vi "CloseConnection.vi"(8 "error in (no error)":errorcluster, 10 "timeout [ms]":i32=5000, 11 "Communicator in":refnum<class "Communicator.lvclass">) -> (0 "error out":errorcluster, 3 "Communicator out":refnum<class "Communicator.lvclass">)   [LabVIEW 2023, in "Communicator.lvclass"]
uses:
  Communicator.lvclass
  Communicator.lvclass/Communicator.ctl
  <vilib>/MediaMongrels Ltd/WebSockets/WebSockets/WebSocket Client/WebSocket Client.lvclass
panel:
  # "Connector Pane"
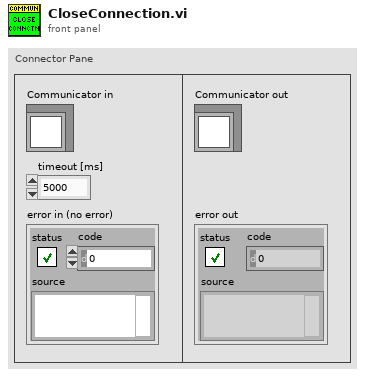
[diagram p1: front panel]
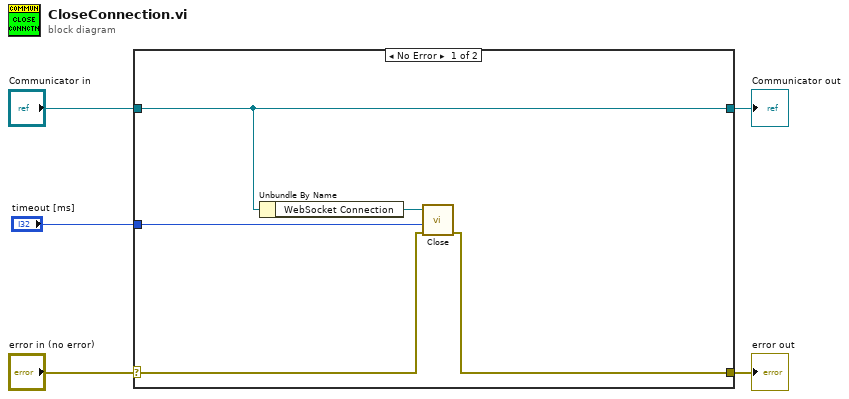
[diagram p0: block diagram]
diagram:
  n1 = case shown="No Error" "error in (no error)" {
    selector: "error in (no error)" -> [w10 w12]
    tunnel: [w9 w12] -> w4
    tunnel: [w8 w11] -> w2
    tunnel: "Communicator in" -> [w8 w11]
    tunnel: "timeout [ms]" -> [w6 _]
    frame No Error {
      n2 = Unbundle By Name(w8) -> ("WebSocket Connection"=w7:refnum<class "WebSocket Client.lvclass">)
      n3 = call-dynamic "Close.vi"("error in (no error)"=w10, "timeout ms (5000)"=w6, "WebSocket in"=w7) -> ("error out"=w9:errorcluster)  [unwired: 8 in]
    }
    frame Error {
    }
  }
  "error out" <- w4
  "Communicator out" <- w2
